vi "UpdateIndicators.vi"() -> (4 "Scanning":bool, 6 "Camera":bool, 9 "andortemperatur":bool, 11 "Interlock":bool, 21 "Mirror":bool, 22 "Scanner":bool, 23 "Online":bool, 24 "AOTF":bool, 25 "Laser":bool caption="seed laser", 26 "Progress":dbl, 27 "temperatureCamera":i32(slide) scale=-100.0..20.0)   [LabVIEW 2011]
uses:
  Variables/GlobalGetCamerasOnOff.vi
  Variables/GlobalGetPhysikalInstrumentsOnOff.vi
  Variables/GlobalGetAOTFOnOff.vi
  Variables/GlobalGetKoherasLaserOnOff.vi
  Variables/GlobalLaserEmissionOnOffInterlook.vi
  Variables/GlobalGetTemperatureCamera.vi
  Variables/GlobalGetMesaurementStatus.vi
  Variables/GlobalSetGetPixelOfRoi.vi
  Variables/GlobalScanningPositionInPixelValues.vi
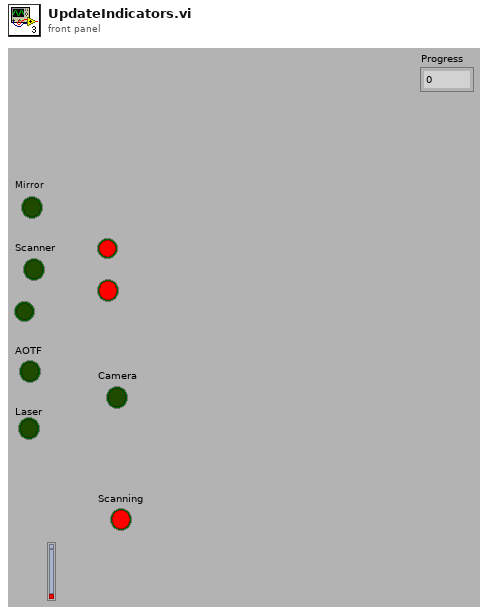
[diagram p1: front panel]
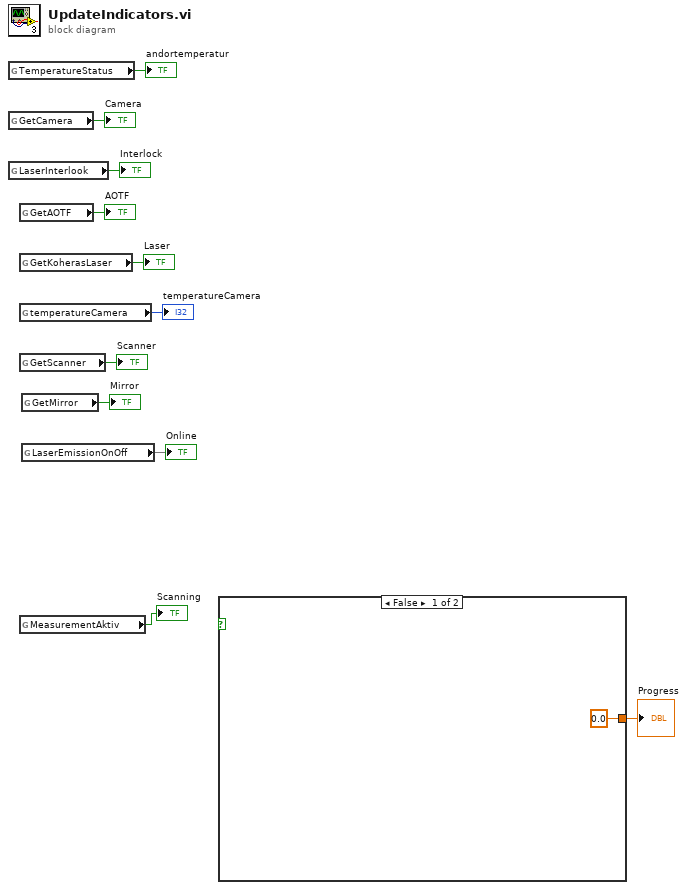
[diagram p0: block diagram]
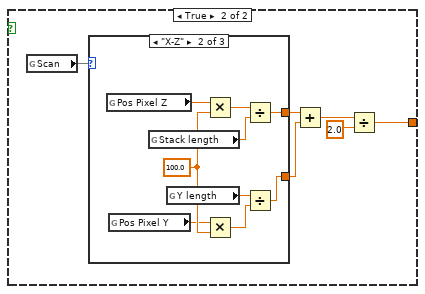
[diagram p2: hidden frame]
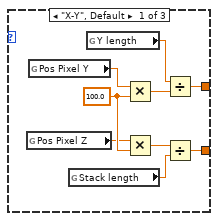
[diagram p3: hidden frame]
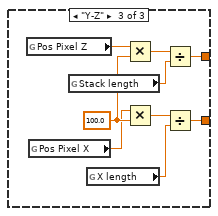
[diagram p4: hidden frame]
diagram:
  n1 = global read "GlobalGetTemperatureCamera.vi" "TemperatureStatus"() -> (→"andortemperatur":bool)
  n2 = global read "GlobalGetCamerasOnOff.vi" "GetCamera"() -> (→"Camera":bool)
  n3 = global read "GlobalLaserEmissionOnOffInterlook.vi" "LaserInterlook"() -> (→"Interlock":bool)
  n4 = global read "GlobalGetAOTFOnOff.vi" "GetAOTF"() -> (→"AOTF":bool)
  n5 = global read "GlobalGetKoherasLaserOnOff.vi" "GetKoherasLaser"() -> (→"Laser":bool)
  n6 = global read "GlobalGetTemperatureCamera.vi" "temperatureCamera"() -> (→"temperatureCamera":i32)
  n7 = global read "GlobalGetPhysikalInstrumentsOnOff.vi" "GetScanner"() -> (→"Scanner":bool)
  n8 = global read "GlobalGetMesaurementStatus.vi" "MeasurementAktiv"() -> (→"Scanning":bool)
  n9 = global read "GlobalGetPhysikalInstrumentsOnOff.vi" "GetMirror"() -> (→"Mirror":bool)
  n10 = global read "GlobalLaserEmissionOnOffInterlook.vi" "LaserEmissionOnOff"() -> (→"Online")
  n11 = case shown="False" {
    selector: _ -> [_ _]
    tunnel: [0.0 w13] -> w1
    frame False {
    }
    frame True {
      n12 = global read "GlobalSetGetPixelOfRoi.vi" "Scan"() -> (w18)
      n13 = case shown="\"X-Z\"" w18 {
        tunnel: [w20 w29 w37] -> w17
        tunnel: [w19 w28 w38] -> w16
        frame "X-Y", Default {
          w27 = 100.0 ("y")
          n14 = global read "GlobalScanningPositionInPixelValues.vi" "Pos Pixel Z"() -> (w25:dbl)
          n15 = global read "GlobalScanningPositionInPixelValues.vi" "Pos Pixel Y"() -> (w23:dbl)
          n16 = global read "GlobalSetGetPixelOfRoi.vi" "Stack length"() -> (w24:dbl)
          n17 = global read "GlobalSetGetPixelOfRoi.vi" "Y length"() -> (w21:dbl)
          n18 = Multiply(x=w23, y=w27) -> (x*y=w22:dbl)
          n19 = Multiply(x=w25, y=w27) -> (x*y=w26:dbl)
          n20 = Divide(x=w21, y=w22) -> (x/y=w20:dbl)
          n21 = Divide(x=w26, y=w24) -> (x/y=w19:dbl)
        }
        frame "X-Z" {
          w36 = 100.0 ("y")
          n22 = global read "GlobalScanningPositionInPixelValues.vi" "Pos Pixel Z"() -> (w34:dbl)
          n23 = global read "GlobalScanningPositionInPixelValues.vi" "Pos Pixel Y"() -> (w32:dbl)
          n24 = global read "GlobalSetGetPixelOfRoi.vi" "Stack length"() -> (w33:dbl)
          n25 = global read "GlobalSetGetPixelOfRoi.vi" "Y length"() -> (w30:dbl)
          n26 = Multiply(x=w34, y=w36) -> (x*y=w35:dbl)
          n27 = Multiply(x=w32, y=w36) -> (x*y=w31:dbl)
          n28 = Divide(x=w35, y=w33) -> (x/y=w29:dbl)
          n29 = Divide(x=w30, y=w31) -> (x/y=w28:dbl)
        }
        frame "Y-Z" {
          w45 = 100.0 ("y")
          n30 = global read "GlobalScanningPositionInPixelValues.vi" "Pos Pixel Z"() -> (w43:dbl)
          n31 = global read "GlobalScanningPositionInPixelValues.vi" "Pos Pixel X"() -> (w40:dbl)
          n32 = global read "GlobalSetGetPixelOfRoi.vi" "Stack length"() -> (w42:dbl)
          n33 = global read "GlobalSetGetPixelOfRoi.vi" "X length"() -> (w39:dbl)
          n34 = Multiply(x=w43, y=w45) -> (x*y=w44:dbl)
          n35 = Multiply(x=w40, y=w45) -> (x*y=w41:dbl)
          n36 = Divide(x=w44, y=w42) -> (x/y=w37:dbl)
          n37 = Divide(x=w41, y=w39) -> (x/y=w38:dbl)
        }
      }
      n38 = Add(x=w17, y=w16) -> (x+y=w15:dbl)
      n39 = Divide(x=w15, y=2.0) -> (x/y=w13:dbl)
    }
  }
  "Progress" <- w1
